vi "Force Sensing-Basic.vi"() -> ()   [LabVIEW 2010]
uses:
  <vilib>/Analysis/Matrix/Datatypes/RealMatrix.ctl
  <vilib>/Utility/file.llb/Write To Spreadsheet File (string).vi
  <vilib>/Analysis/_algsub.llb/Real PseudoInverse Matrix.vi
  <vilib>/Analysis/baseanly.llb/Real A x B.vi
  <vilib>/Analysis/_algsub.llb/Real Vector Norm.vi
  <vilib>/Analysis/NI_AALPro.lvlib
  <vilib>/Analysis/NI_AALBase.lvlib
  <vilib>/Analysis/Matrix/NI_Matrix.lvlib
panel:
  in  "stop":bool
  in  "Force Scaling Factor":dbl=1.0
  in  "Record Switch":bool
  in  "file path (dialog if empty)":path=path "C:/Users/Berk/Desktop/closed_washer0_1"
  out "Measured Tip Forces [mN]":u8(slide) scale=0.0..10.0
  in  "Plot Switch":bool
  out "Ftotal [mN]":dbl format="%.1f"
  out "Fy [mN]":dbl format="%.1f"
  out "Fx [mN]":dbl format="%.1f"
  in  "sm130 IP Address":string="192.168.0.11"
  in  "Rebias":bool
  out "Active Calibration Matrix":dbl[][](array[numeric])
  in  "Select Your Tool":T1(radio)=enum."2 DOF MicroNeedle"
  out "Shift 3":dbl format="%.3f"
  out "Shift 2":dbl format="%.3f"
  out "Shift 1":dbl format="%.3f"
  out "Channel 3":dbl format="%.3g"
  out "Channel 2":dbl format="%.3g"
  out "Channel 1":dbl format="%#.3g"
  out "Average 3":dbl format="%.3g"
  out "Average 2":dbl format="%.3g"
  out "Average 1":dbl format="%.3g"
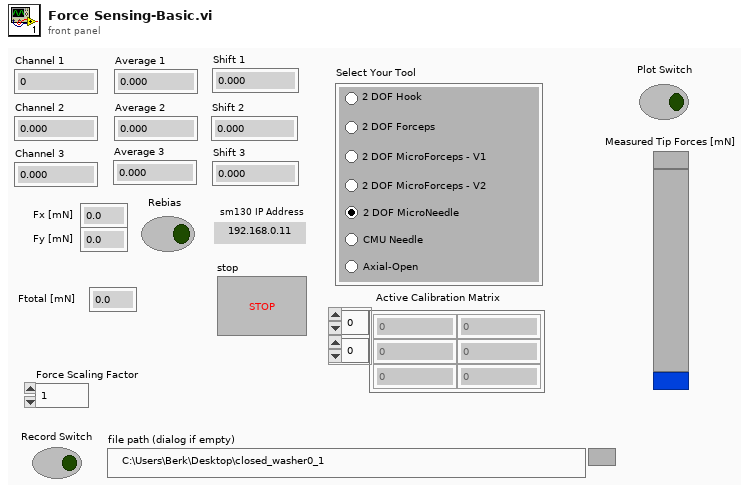
[diagram p1: front panel]
types:
  T1 = enum32{"2 DOF Hook", "2 DOF Forceps", "2 DOF MicroForceps - V1", "2 DOF MicroForceps - V2", "2 DOF MicroNeedle", "CMU Needle", "Axial-Open"}
  T2 = typedef "NI_Matrix.lvlib/RealMatrix.ctl" = dbl[][]
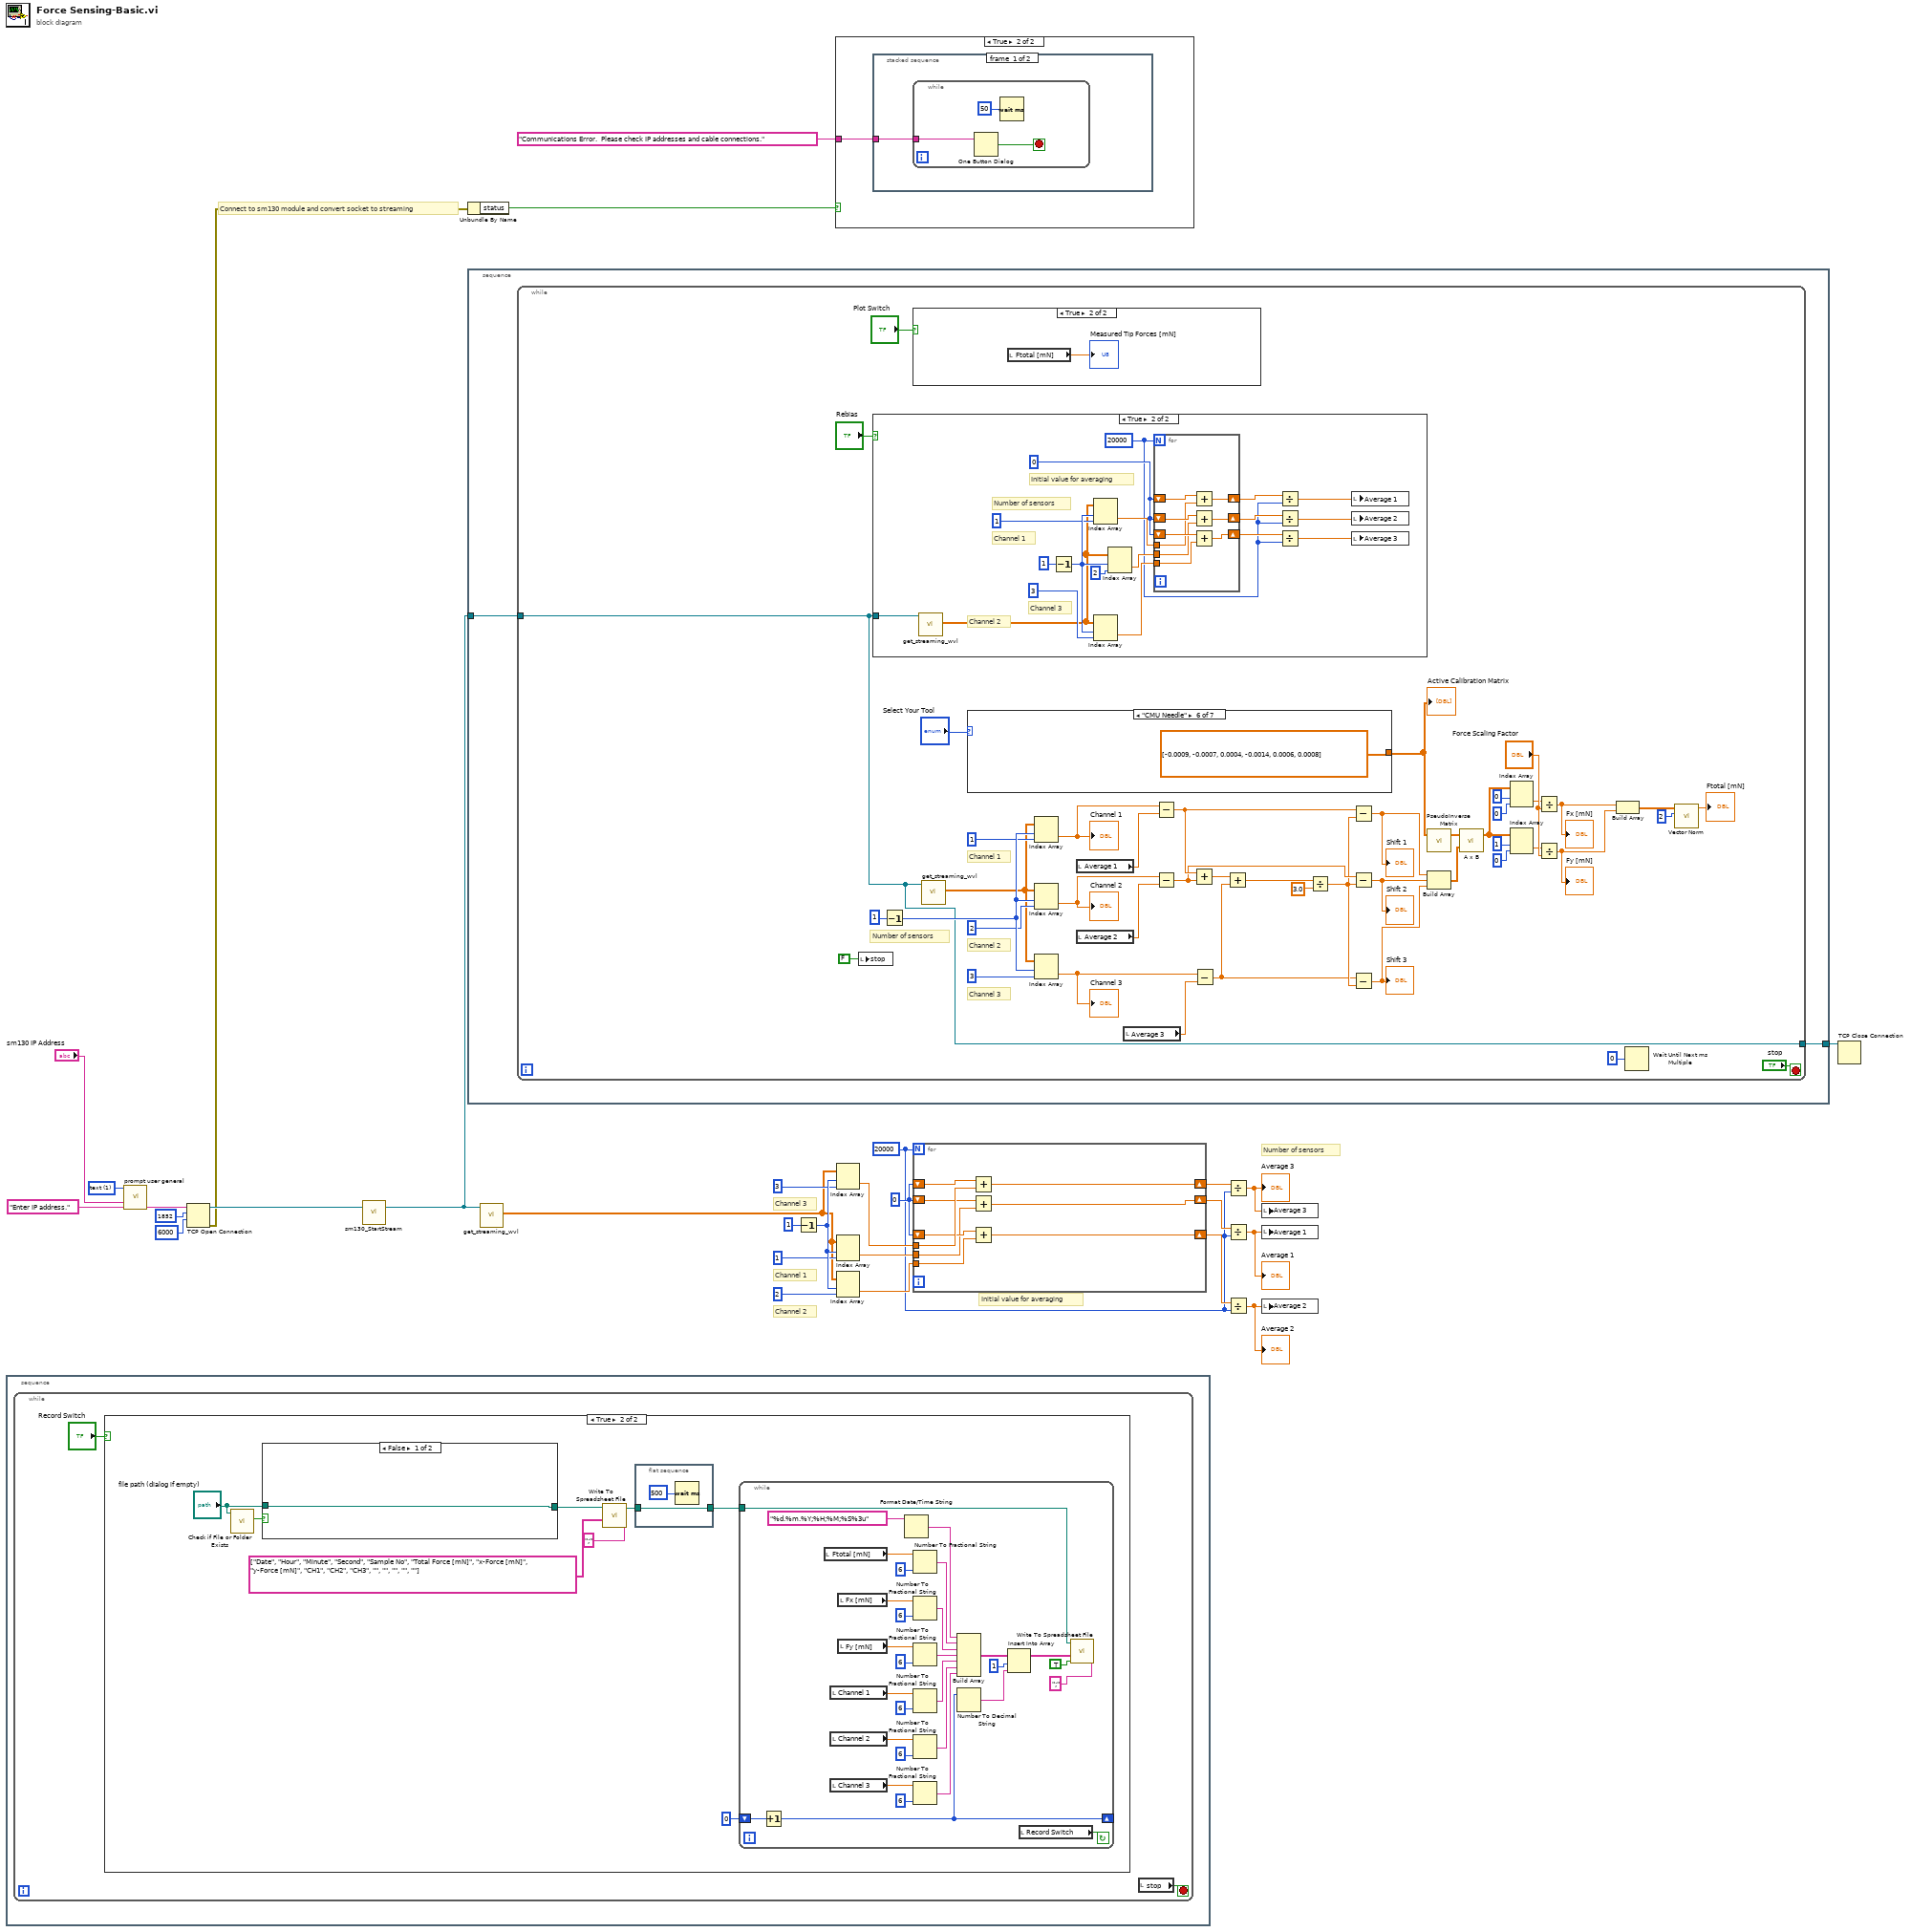
[diagram p0: block diagram]
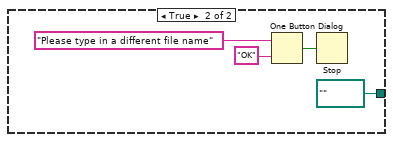
[diagram p3: hidden frame]
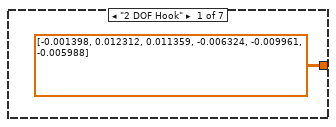
[diagram p6: hidden frame]
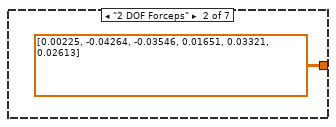
[diagram p7: hidden frame]
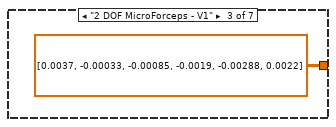
[diagram p8: hidden frame]
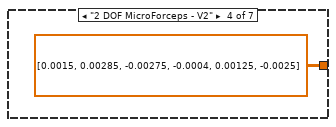
[diagram p9: hidden frame]
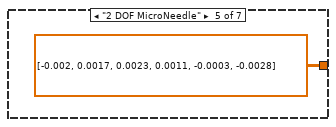
[diagram p10: hidden frame]
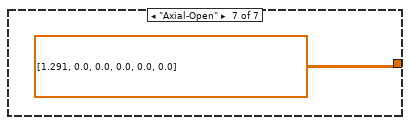
[diagram p11: hidden frame]
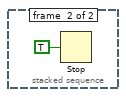
[diagram p13: hidden frame]
diagram:
  w4 = 20000
  w5 = 0
  w26 = u16 1 items=["numeric", "text"] ("control type")
  # "Initial value for averaging"
  # "Channel 3"
  # "Channel 2"
  # "Channel 1"
  # "Number of sensors"
  # "Connect to sm130 module and convert socket to streaming"
  n1 = stacked-sequence {
    frame #0 {
      n2 = while {
        stop <- w30 stop-if-true
        n3 = case shown="True" "Record Switch" {
          frame False {
          }
          frame True {
            n4 = call <vilib>:"Check if File or Folder Exists.vi"("path"="file path (dialog if empty)") -> ("file or folder exists?"=w36:bool)  [unwired: 8 in, 2 out]
            n5 = case shown="False" w36 {
              tunnel: [w70 path "" ("file path (dialog if empty)")] -> w37
              tunnel: "file path (dialog if empty)" -> [w70 _]
              frame False {
              }
              frame True {
                n6 = One Button Dialog(message="Please type in a different file name", button name ("OK")="OK") -> (true=w72:bool)
                n7 = Stop(stop? (T)=w72) -> ()
              }
            }
            n8 = call-poly <vilib>:"Write To Spreadsheet File.vi"("delimiter (\\t)"=";" ("delimiter (\\t)"), "1D data"=string[] ["Date", "Hour", "Minute", "Second", "Sample No", "Total Force [mN]", "x-Force [mN]", "y-Force [mN]", "CH1", "CH2", "CH3", "", "", "", "", ""], "file path (dialog if empty)"=w37) -> ("new file path (Not A Path if cancelled)"=w34:path)  [unwired: 5 in]
            n9 = flat-sequence {
              tunnel: [w75] -> w33
              tunnel: w34 -> [w75]
              frame #0 {
                n10 = Wait (ms)(milliseconds to wait=u32 500) -> ()  [unwired: 1 out]
              }
            }
            n11 = while {
              shift-right: [w62] -> _
              shift-left: 0 -> [w51]
              tunnel: w33 -> [w50]
              stop <- w43 continue-if-true
              n12 = Increment(x=w51) -> (x+1=w62:i32)
              n13 = local read "Ftotal [mN]"() -> (w58:dbl)
              n14 = local read "Channel 1"() -> (w45:dbl)
              n15 = local read "Channel 2"() -> (w46:dbl)
              n16 = local read "Channel 3"() -> (w44:dbl)
              n17 = local read "Fx [mN]"() -> (w55:dbl)
              n18 = local read "Fy [mN]"() -> (w54:dbl)
              n19 = Format Date/Time String(time format string (%c)="%d.%m.%Y;%H;%M;%S%3u") -> (date/time string=w68:string)  [unwired: 2 in]
              n20 = Number To Fractional String(number=w58, precision (6)=i16 6) -> (F-format string=w66:string)  [unwired: 2 in]
              n21 = Number To Fractional String(number=w55, precision (6)=i16 6) -> (F-format string=w53:string)  [unwired: 2 in]
              n22 = Number To Fractional String(number=w54, precision (6)=i16 6) -> (F-format string=w52:string)  [unwired: 2 in]
              n23 = Number To Fractional String(number=w45, precision (6)=i16 6) -> (F-format string=w42:string)  [unwired: 2 in]
              n24 = Number To Fractional String(number=w46, precision (6)=i16 6) -> (F-format string=w41:string)  [unwired: 2 in]
              n25 = Number To Fractional String(number=w44, precision (6)=i16 6) -> (F-format string=w40:string)  [unwired: 2 in]
              n26 = Build Array(w68, w66, w53, w52, w42, w41, w40) -> (w65:string[])
              n27 = Number To Decimal String(number=w62) -> (decimal integer string=w63:string)  [unwired: 1 in]
              n28 = Insert Into Array(array=w65, index=1, new element=w63) -> (w61:string[])
              n29 = local read "Record Switch"() -> (w43:bool)
              n30 = call-poly <vilib>:"Write To Spreadsheet File.vi"("delimiter (\\t)"=";" ("delimiter (\\t)"), "append to file? (new file:F)"=TRUE, "1D data"=w61, "file path (dialog if empty)"=w50) -> ()  [unwired: 4 in, 1 out]
            }
          }
        }
        n31 = local read "stop"() -> (w30:bool)
      }
    }
  }
  n32 = call "prompt user general.vi"("control type"=w26, "text default"="sm130 IP Address", "message to display"="Enter IP address.") -> ("Text output"=w20:string)  [unwired: 11 in, 1 out]
  n33 = TCP Open Connection(address=w20, remote port or service name=u16 1852 ("remote port"), timeout ms (60000)=6000) -> (connection ID=w25:refnum<k5>, error out=w22:errorcluster)  [unwired: 2 in]
  n34 = call "sm130_StartStream.vi"("Connection ID In"=w25) -> ("Stream ID Out"=w28:refnum<k5>)  [unwired: 1 in, 1 out]
  n35 = Unbundle By Name(w22) -> ("status"=w21:bool)
  n36 = stacked-sequence {
    tunnel: w28 -> [w78]
    tunnel: [w77] -> w29
    frame #0 {
      n37 = while {
        tunnel: [w112] -> w77
        tunnel: w78 -> [w112]
        stop <- "stop" stop-if-true
        # "Channel 3"
        # "Channel 2"
        # "Channel 1"
        # "Number of sensors"
        n38 = local write "stop"(FALSE) -> ()
        n39 = case shown="True" "Rebias" {
          tunnel: w112 -> [_ w142]
          frame False {
          }
          frame True {
            w129 = 0
            w128 = 20000
            # "Initial value for averaging"
            # "Channel 3"
            # "Channel 2"
            # "Channel 1"
            # "Number of sensors"
            n40 = call "get_streaming_wvl.vi"("Stream ID Out"=w142) -> ("Array"=w136:dbl[][])  [unwired: 9 in, 1 out]
            n41 = Decrement(x=1) -> (x-1=w140:i32)
            n42 = Index Array(array=w136, index (row)=w140, index (col)=1) -> (element=w133:dbl)
            n43 = Index Array(array=w136, index (row)=w140, index (col)=3) -> (element=w135:dbl)
            n44 = Index Array(array=w136, index (row)=w140, index (col)=2) -> (element=w134:dbl)
            n45 = for {
              N: w128 -> [_]
              shift-right: [w145] -> w132
              shift-left: w129 -> [w144]
              shift-right: [w146] -> w131
              shift-left: w129 -> [w147]
              shift-right: [w151] -> w130
              shift-left: w129 -> [w149]
              tunnel: w135 -> [w150]
              tunnel: w134 -> [w148]
              tunnel: w133 -> [w143]
              n46 = Add(x=w144, y=w143) -> (x+y=w145:dbl)
              n47 = Add(x=w147, y=w148) -> (x+y=w146:dbl)
              n48 = Add(x=w149, y=w150) -> (x+y=w151:dbl)
            }
            n49 = Divide(x=w132, y=w128) -> (x/y=w127:dbl)
            n50 = Divide(x=w131, y=w128) -> (x/y=w126:dbl)
            n51 = Divide(x=w130, y=w128) -> (x/y=w125:dbl)
            n52 = local write "Average 1"(w127) -> ()
            n53 = local write "Average 2"(w126) -> ()
            n54 = local write "Average 3"(w125) -> ()
          }
        }
        n55 = Decrement(x=1) -> (x-1=w122:i32)
        n56 = case shown="True" "Plot Switch" {
          frame False {
          }
          frame True {
            n57 = local read "Ftotal [mN]"() -> (→"Measured Tip Forces [mN]":dbl)
          }
        }
        n58 = call "get_streaming_wvl.vi"("Stream ID Out"=w112) -> ("Array"=w118:dbl[][])  [unwired: 9 in, 1 out]
        n59 = case shown="\"CMU Needle\"" "Select Your Tool" {
          tunnel: [T2 [[-0.001398, 0.012312], [0.011359, -0.006324], [-0.009961, -0.005988]] ("output matrix") T2 [[0.00225, -0.04264], [-0.03546, 0.01651], [0.03321, 0.02613]] ("output matrix") T2 [[0.0037, -0.00033], [-0.00085, -0.0019], [-0.00288, 0.0022]] ("output matrix") T2 [[0.0015, 0.00285], [-0.00275, -0.0004], [0.00125, -0.0025]] ("output matrix") T2 [[-0.002, 0.0017], [0.0023, 0.0011], [-0.0003, -0.0028]] ("output matrix") T2 [[-0.0009, -0.0007], [0.0004, -0.0014], [0.0006, 0.0008]] ("output matrix") T2 [[1.291, 0.0], [0.0, 0.0], [0.0, 0.0]] ("output matrix")] -> w110
          frame "2 DOF Hook" {
          }
          frame "2 DOF Forceps" {
          }
          frame "2 DOF MicroForceps - V1" {
          }
          frame "2 DOF MicroForceps - V2" {
          }
          frame "2 DOF MicroNeedle" {
          }
          frame "CMU Needle" {
          }
          frame "Axial-Open" {
          }
        }
        "Active Calibration Matrix" <- w110
        n60 = Index Array(array=w118, index (row)=w122, index (col)=1) -> (element=w83:dbl)
        "Channel 1" <- w83
        n61 = Index Array(array=w118, index (row)=w122, index (col)=2) -> (element=w85:dbl)
        "Channel 2" <- w85
        n62 = Index Array(array=w118, index (row)=w122, index (col)=3) -> (element=w84:dbl)
        "Channel 3" <- w84
        n63 = local read "Average 1"() -> (w114:dbl)
        n64 = local read "Average 2"() -> (w113:dbl)
        n65 = local read "Average 3"() -> (w115:dbl)
        n66 = Subtract(x=w83, y=w114) -> (x-y=w94:dbl)
        n67 = Subtract(x=w85, y=w113) -> (x-y=w93:dbl)
        n68 = Add(x=w94, y=w93) -> (x+y=w97:dbl)
        n69 = Subtract(x=w84, y=w115) -> (x-y=w91:dbl)
        n70 = Add(x=w97, y=w91) -> (x+y=w96:dbl)
        n71 = Divide(x=w96, y=3.0) -> (x/y=w92:dbl)
        n72 = Subtract(x=w94, y=w92) -> (x-y=w88:dbl)
        "Shift 1" <- w88
        n73 = Subtract(x=w93, y=w92) -> (x-y=w89:dbl)
        "Shift 2" <- w89
        n74 = Subtract(x=w91, y=w92) -> (x-y=w90:dbl)
        "Shift 3" <- w90
        n75 = call-poly <vilib>:"PseudoInverse Matrix.vi"("Input Matrix"=w110) -> ("PseudoInverse Matrix"=w117:T2)  [unwired: 1 in, 1 out]
        n76 = Build Array ("Build Matrix")(w88, w89, w90) -> (w116:T2)
        n77 = call-poly <vilib>:"A x B.vi"("B"=w116, "A"=w117) -> ("A x B"=w108:T2)  [unwired: 1 out]
        n78 = Index Array(array=w108, index (row)=0, index (col)=0 ("index (row)")) -> (element=w82:dbl)
        n79 = Index Array(array=w108, index (row)=1, index (col)=0 ("index (row)")) -> (element=w81:dbl)
        n80 = Divide(x=w82, y="Force Scaling Factor") -> (x/y=w87:dbl)
        "Fx [mN]" <- w87
        n81 = Divide(x=w81, y="Force Scaling Factor") -> (x/y=w86:dbl)
        "Fy [mN]" <- w86
        n82 = Build Array(w87, w86) -> (w101:dbl[])
        n83 = Wait Until Next ms Multiple(millisecond multiple=0) -> ()  [unwired: 1 out]
        n84 = call-poly <vilib>:"Vector Norm.vi"("norm type"=2, "Input Vector"=w101) -> ("norm"=→"Ftotal [mN]":dbl)  [unwired: 8 in, 1 out]
      }
    }
  }
  n85 = call "get_streaming_wvl.vi"("Stream ID Out"=w28) -> ("Array"=w12:dbl[][])  [unwired: 9 in, 1 out]
  n86 = Decrement(x=1) -> (x-1=w16:i32)
  n87 = case shown="True" w21 {
    tunnel: "Communications Error.  Please check IP addresses and cable connections." ("message") -> [_ w159]
    frame False {
    }
    frame True {
      n88 = stacked-sequence {
        tunnel: w159 -> [w160 _]
        frame #0 {
          n89 = while {
            tunnel: w160 -> [w161]
            stop <- w163 stop-if-true
            n90 = One Button Dialog(message=w161) -> (true=w163:bool)  [unwired: 1 in]
            n91 = Wait (ms)(milliseconds to wait=u32 50) -> ()  [unwired: 1 out]
          }
        }
        frame #1 {
          n92 = Stop(stop? (T)=TRUE) -> ()
        }
      }
    }
  }
  n93 = Index Array(array=w12, index (row)=w16, index (col)=3) -> (element=w11:dbl)
  n94 = Index Array(array=w12, index (row)=w16, index (col)=1) -> (element=w9:dbl)
  n95 = Index Array(array=w12, index (row)=w16, index (col)=2) -> (element=w10:dbl)
  n96 = for {
    N: w4 -> [_]
    shift-right: [w167] -> w8
    shift-left: w5 -> [w166]
    shift-right: [w168] -> w7
    shift-left: w5 -> [w169]
    shift-right: [w173] -> w6
    shift-left: w5 -> [w171]
    tunnel: w11 -> [w172]
    tunnel: w10 -> [w170]
    tunnel: w9 -> [w165]
    n97 = Add(x=w171, y=w172) -> (x+y=w173:dbl)
    n98 = Add(x=w166, y=w165) -> (x+y=w167:dbl)
    n99 = Add(x=w169, y=w170) -> (x+y=w168:dbl)
  }
  n100 = Divide(x=w6, y=w4) -> (x/y=w1:dbl)
  "Average 3" <- w1
  n101 = Divide(x=w8, y=w4) -> (x/y=w3:dbl)
  "Average 1" <- w3
  n102 = Divide(x=w7, y=w4) -> (x/y=w2:dbl)
  "Average 2" <- w2
  n103 = local write "Average 3"(w1) -> ()
  n104 = local write "Average 1"(w3) -> ()
  n105 = local write "Average 2"(w2) -> ()
  n106 = TCP Close Connection(connection ID=w29) -> ()  [unwired: 2 in, 2 out]
